vi "TW Fix VI Missing Paths by Directory.vi"(8 "error in (no error)":errorcluster, 9 "New Subname":string, 10 "Subname to Replace":string, 11 "Folder Path":path) -> (0 "error out":errorcluster)   [LabVIEW 2021]
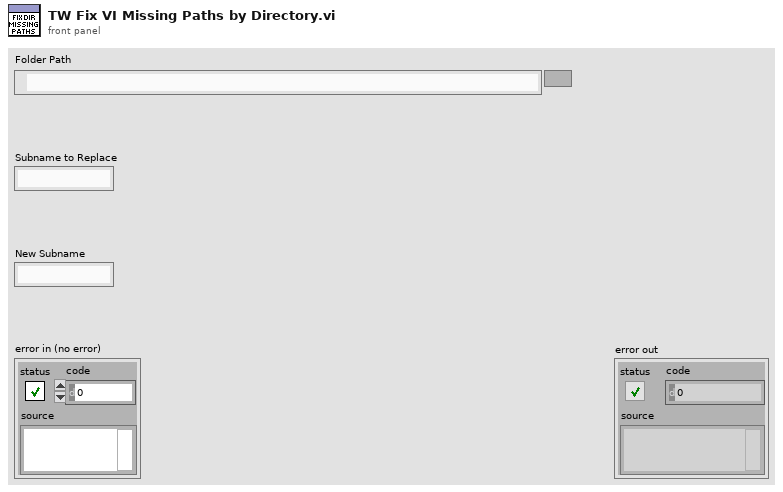
[diagram p1: front panel]
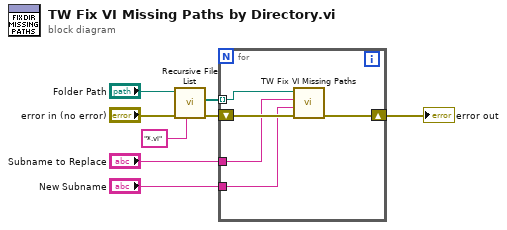
[diagram p0: block diagram]
diagram:
  n1 = call <vilib>:"Recursive File List.vi"("pattern"="*.vi", "error in (no error)"="error in (no error)", "Folder Path"="Folder Path") -> ("error out"=w6:errorcluster, "All Files in Dir"=w8:path[])  [unwired: 4 in, 3 out]
  n2 = for {
    tunnel: w8 -> [w13] mode=indexing
    shift-right: [w12] -> w4
    shift-left: w6 -> [w11]
    tunnel: "Subname to Replace" -> [w10]
    tunnel: "New Subname" -> [w9]
    n3 = call "TW Fix VI Missing Paths.vi"("error in (no error)"=w11, "New Subname"=w9, "Subname to Replace"=w10, "VI Path"=w13) -> ("error out"=w12:errorcluster)  [unwired: 7 in]
  }
  "error out" <- w4
